vi "WithParent_TreeHasItem.vi"() -> (0 "error out":errorcluster)   [LabVIEW 2017, in "ResultTree.Tests.lvlib" / "AddTestCase.lvlib"]
uses:
  AddTestCase.lvlib
  c09b0184-a7a5-4658-999a-d2ef6d2e958d.vi
  Constraint/IsEqual/Create.vi
  Constraint/IsEqual/IsEqual.lvclass
  ResultTree/ResultTree.lvclass
panel:
  in  "Tree":string(tree)
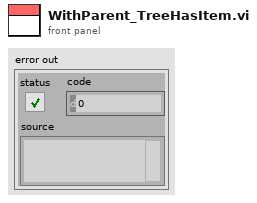
[diagram p1: front panel]
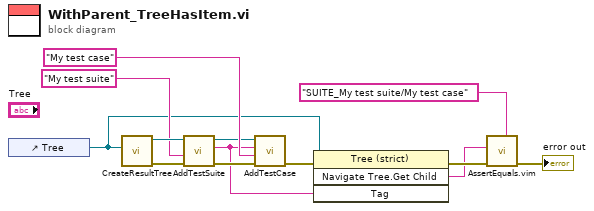
[diagram p0: block diagram]
diagram:
  n1 = control-ref of="Tree"() -> (w3:refnum<vi>)
  n2 = call "CreateResultTree.vi"("Tree Refnum"=w3) -> ("error out"=w12:errorcluster, "ResultTree out"=w8:refnum<class "ResultTree.lvclass">)  [unwired: 9 in]
  n3 = call "AddTestSuite.vi"("error in (no error)"=w12, "Name"="My test suite", "ResultTree in"=w8) -> ("error out"=w9:errorcluster, "Tag Name"=w2:string, "ResultTree out"=w7:refnum<class "ResultTree.lvclass">)  [unwired: 6 in]
  n4 = call "AddTestCase.vi"("error in (no error)"=w9, "Name"="My test case", "Parent Tag (\"\")"=w2, "ResultTree in"=w7) -> ("error out"=w5:errorcluster)  [unwired: 5 in, 2 out]
  n5 = invoke class="Tree (strict)" method="Navigate Tree.Get Child"(reference=w3, error in=w5, "Tag"=w2) -> (error out=w4:errorcluster, "Navigate Tree:Get Child"=w1:string)  [unwired: 1 in, 2 out]
  n6 = call "AssertEquals.vim"("Expected"="SUITE_My test suite/My test case" ("Name"), "error in (no error)"=w4, "Actual"=w1) -> ("error out"=→"error out":errorcluster)  [unwired: 8 in]
